vi "checkAddressee.vi"(0 "Host_Reference":refnum<class "HGF_Reference.lvclass">, 2 "MoAgSy_Message":refnum<class "MoAgSy_Message.lvclass">, 5 "error in (no error)":errorcluster) -> (10 "addressee":string, 14 "dup HGF_Reference":refnum<class "HGF_Reference.lvclass">, 16 "dup MoAgSy_Message":refnum<class "MoAgSy_Message.lvclass">, 17 "Destination":string, 18 "receiver":T1(ring), 19 "error out":errorcluster)   [LabVIEW 2009, in "MoAgSy.lvlib" / "MoAgSy_Host.lvclass"]
doc: "<B>public</B> VI checks addressee of incoming messages.\n\nF.Berck@gsi.de\nGSI Darmstadt 2009"
uses:
  MoAgSy_Host.lvclass
  MoAgSy_Message/MoAgSy_Message.lvclass
  HGF_BaseClasses/HGF_Reference/HGF_Reference.lvclass
panel:
  in  "timeout in ms (-1)":i32
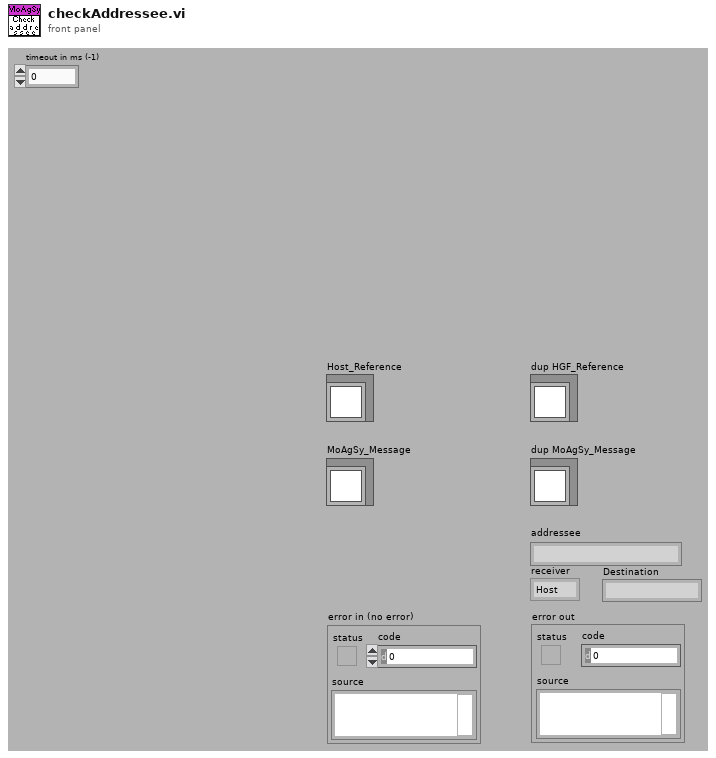
[diagram p1: front panel]
types:
  T1 = enum16{"Host", "running agent", "past Agent", "unknown"}
  T2 = cluster{"Host Name":string, "Maximum number of running Agents":i16, "ID":string}
  T3 = cluster{"Agent ID":string, "Destination":string}[]
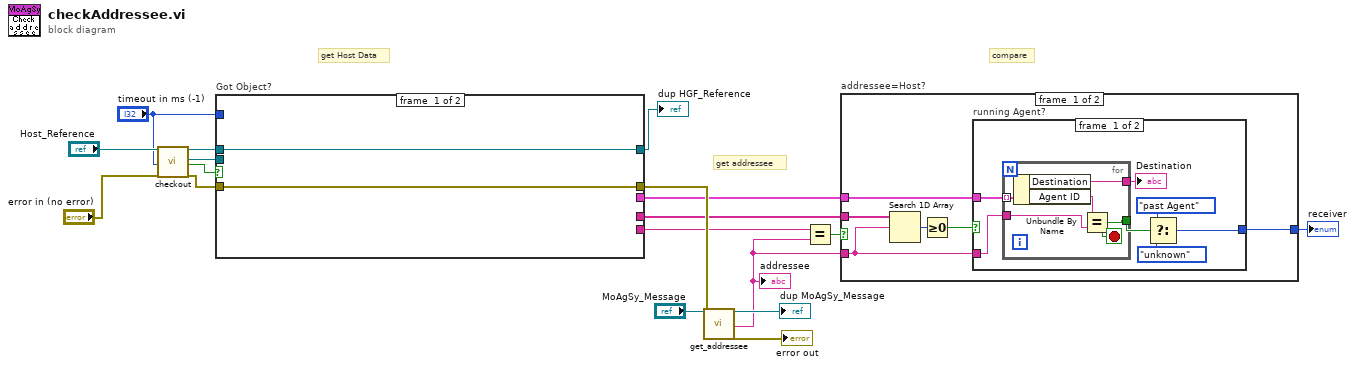
[diagram p0: block diagram]
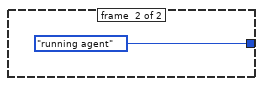
[diagram p2: hidden frame]
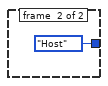
[diagram p3: hidden frame]
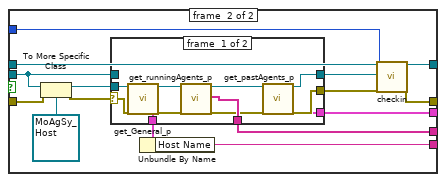
[diagram p4: hidden frame]
diagram:
  # "compare"
  # "get addressee"
  # "get Host Data"
  n1 = call "checkout.vi"("HGF_Reference"="Host_Reference", "timeout in ms (-1)"="timeout in ms (-1)", "error in (no error)"="error in (no error)") -> ("dup HGF_Reference"=w14:refnum<class "HGF_Reference.lvclass">, "Object"=w13:refnum<class>, "got object?"=w12:bool, "error out"=w11:errorcluster)  [unwired: 13 out]
  n2 = case "Got Object?" shown="True" w12 {
    tunnel: w11 -> [w19 w35]
    tunnel: w13 -> [_ w26]
    tunnel: w14 -> [w20 w33]
    tunnel: [w20 w32] -> w10
    tunnel: "timeout in ms (-1)" -> [_ w31]
    tunnel: [w19 w30] -> w7
    tunnel: [_ w24] -> w5
    tunnel: [_ w22] -> w3
    tunnel: [_ w21] -> w1
    frame #0 {
    }
    frame #1 {
      n3 = To More Specific Class(target class=refnum<class "MoAgSy_Host.lvclass"> refnum ("MoAgSy.lvlib:MoAgSy_Host.lvclass"), reference=w26, error in=w35) -> (specific class reference=w29:refnum<class "MoAgSy_Host.lvclass">, error out=w27:errorcluster)
      n4 = case shown="No Error" w27 {
        selector: w27 -> [w45 w47]
        tunnel: w29 -> [w46 _]
        tunnel: [w37 w48] -> w28
        tunnel: w26 -> [_ w48]
        tunnel: [w44 _] -> w25
        tunnel: [w38 w47] -> w23
        tunnel: [w41 _] -> w22
        tunnel: [w36 _] -> w21
        frame #0 {
          n5 = call "get_General_p.vi"("MoAgSy_Host"=w46, "error in (no error)"=w45) -> ("dup MoAgSy_Host"=w43:refnum<class "MoAgSy_Host.lvclass">, "General"=w44:T2, "error out"=w42:errorcluster)  [unwired: 15 out]
          n6 = call "get_runningAgents_p.vi"("MoAgSy_Host"=w43, "error in (no error)"=w42) -> ("dup MoAgSy_Host"=w40:refnum<class "MoAgSy_Host.lvclass">, "Running Agents"=w41:string[], "error out"=w39:errorcluster)  [unwired: 15 out]
          n7 = call "get_pastAgents_p.vi"("MoAgSy_Host"=w40, "error in (no error)"=w39) -> ("dup MoAgSy_Host"=w37:refnum<class "MoAgSy_Host.lvclass">, "past agents"=w36:T3, "error out"=w38:errorcluster)  [unwired: 15 out]
        }
        frame #1 {
        }
      }
      n8 = Unbundle By Name(w25) -> ("Host Name"=w24:string)
      n9 = call "checkin.vi"("HGF_Reference"=w33, "Object"=w28, "timeout /ms (-1)"=w31, "error in (no error)"=w23) -> ("dup HGF_Reference"=w32:refnum<class "HGF_Reference.lvclass">, "error out"=w30:errorcluster)  [unwired: 14 out]
    }
  }
  "dup HGF_Reference" <- w10
  n10 = call "get_addressee.vi"("MoAgSy_Message in"="MoAgSy_Message", "error in (no error)"=w7) -> ("MoAgSy_Message out"=→"dup MoAgSy_Message":refnum<class "MoAgSy_Message.lvclass">, "addressee"=w4:string, "error out"=→"error out":errorcluster)  [unwired: 15 out]
  "addressee" <- w4
  n11 = Equal?(x=w5, y=w4) -> (x = y?=w6:bool)
  n12 = case "addressee=Host?" shown="True" w6 {
    tunnel: w4 -> [w50 _]
    tunnel: w3 -> [w54 _]
    tunnel: [w51 T1."Host"] -> w2
    tunnel: w1 -> [w49 _]
    frame #0 {
      n13 = Search 1D Array(1D array=w54, element=w50) -> (index of element=w53:i32)  [unwired: 1 out]
      n14 = Greater Or Equal To 0?(x=w53) -> (x >= 0?=w52:bool)
      n15 = case "running Agent?" shown="False" w52 {
        tunnel: [w57 T1."running agent"] -> w51
        tunnel: w50 -> [w60 _]
        tunnel: w49 -> [w61 _]
        frame #0 {
          n16 = for {
            tunnel: w61 -> [w66] mode=indexing
            tunnel: w60 -> [w64]
            tunnel: [w63] -> w59
            tunnel: [w62] -> w58
            stop <- w62 stop-if-true
            n17 = Unbundle By Name(w66) -> ("Destination"=w63:string, "Agent ID"=w65:string)
            n18 = Equal?(x=w65, y=w64) -> (x = y?=w62:bool)
          }
          "Destination" <- w59
          n19 = Select(t=T1."past Agent" ("Enum"), s=w58, f=T1."unknown") -> (s? t:f=w57:T1)
        }
        frame #1 {
        }
      }
    }
    frame #1 {
    }
  }
  "receiver" <- w2
